vi "Library.Get All VIs.vi"(8 "error in (no error)":errorcluster, 11 "library ref":refnum<vi>) -> (0 "error out":errorcluster, 3 "vi refs":refnum<vi>[](array[refnum]))   [LabVIEW 2016, in "Build Automation.lvlib"]
uses:
  Build Automation.lvlib
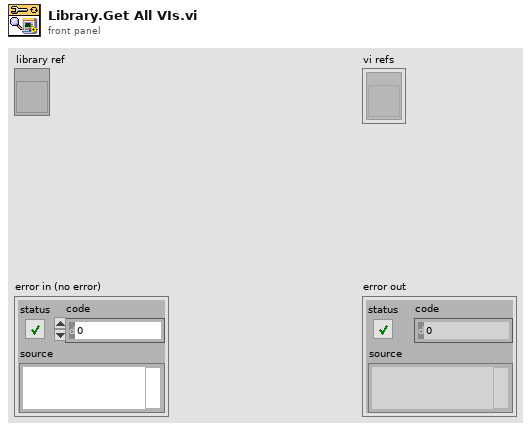
[diagram p1: front panel]
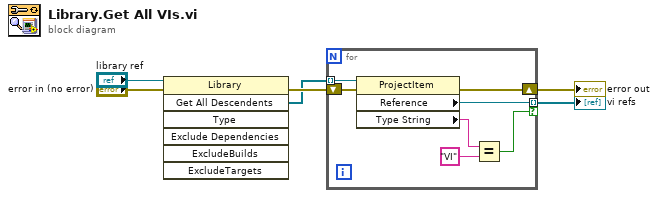
[diagram p0: block diagram]
diagram:
  n1 = invoke class="Library" method="Get All Descendents"(reference="library ref", error in="error in (no error)") -> (error out=w5:errorcluster, "All Descendents"=w4:refnum<vi>[])  [unwired: 5 in, 5 out]
  n2 = for {
    tunnel: w4 -> [w13] mode=indexing
    shift-right: [w10] -> w2
    shift-left: w5 -> [w11]
    tunnel: [w8] -> w1 mode=indexing if=w7
    n3 = property class="ProjectItem"(reference=w13, error in=w11) -> (error out=w10:errorcluster, "Reference"=w8:refnum<vi>, "Type String"=w9:string)  [unwired: 1 out]
    n4 = Equal?(x=w9, y="VI") -> (x = y?=w7:bool)
  }
  "error out" <- w2
  "vi refs" <- w1
